vi "Enqueue Close Connection.vi"(8 "Error In":errorcluster, 11 "Name":string) -> (0 "Error Out":errorcluster)   [LabVIEW 2019, in "SR_2000.lvlib"]
uses:
  SR_2000.lvlib
  Queue/Queue.lvlib
  Data Error Notifier/Data and Error Notifier.lvlib
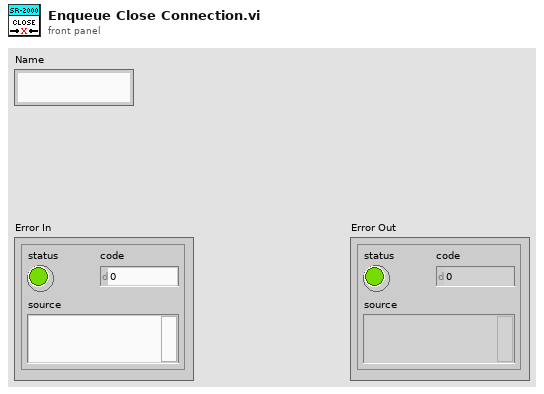
[diagram p1: front panel]
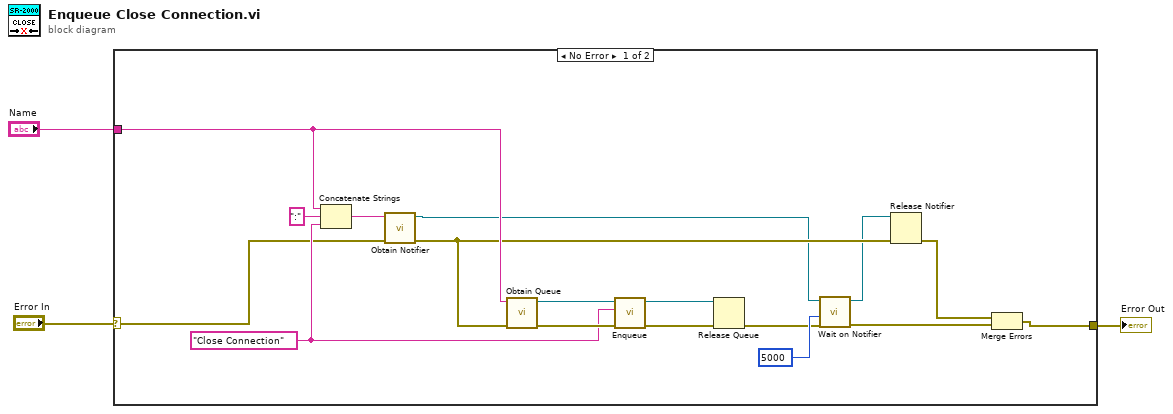
[diagram p0: block diagram]
diagram:
  n1 = case shown="No Error" "Error In" {
    selector: "Error In" -> [w10 w21]
    tunnel: [w12 w21] -> w2
    tunnel: "Name" -> [w19 _]
    frame No Error {
      w17 = "Close Connection" ("Message")
      n2 = Concatenate Strings(w19, ":" ("string"), w17) -> (w11:string)
      n3 = call "Obtain Notifier.vi"("Error In"=w10, "Name"=w11) -> ("Error Out"=w9:errorcluster, "notifier out"=w8:refnum<notifier>)  [unwired: 8 in]
      n4 = call "Obtain Queue.vi"("Error In"=w9, "Name"=w19) -> ("Error Out"=w20:errorcluster, "queue out"=w15:refnum<queue>)  [unwired: 8 in]
      n5 = call "Enqueue.vi"("Error In"=w20, "Message"=w17, "queue in"=w15) -> ("Error Out"=w16:errorcluster, "queue out"=w14:refnum<queue>)  [unwired: 7 in]
      n6 = Release Queue(queue=w14, error in (no error)=w16) -> (error out=w6:errorcluster)  [unwired: 1 in, 2 out]
      n7 = call "Wait on Notifier.vi"("Error In"=w6, "timeout in ms (-1)"=5000, "notifier in"=w8) -> ("Error Out"=w4:errorcluster, "notifier out"=w5:refnum<notifier>)  [unwired: 6 in, 1 out]
      n8 = Release Notifier(notifier=w5, error in (no error)=w9) -> (error out=w13:errorcluster)  [unwired: 1 in, 2 out]
      n9 = Merge Errors(w13, w4) -> (w12:errorcluster)
    }
    frame Error {
    }
  }
  "Error Out" <- w2
